vi "Auto_Routine_StraightTwoPiece.vi"(8 "error in (no error)":errorcluster) -> (0 "error out":errorcluster)   [LabVIEW 2023]
uses:
  Arm2/ArmGetSetpointEnum.ctl
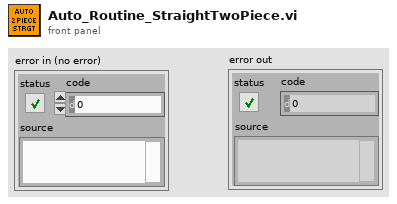
[diagram p1: front panel]
types:
  T1 = typedef "ArmGetSetpointEnum.ctl" = enum16{"ArmFloorPickup", "ArmAmpDeposit", "ArmSpeakerShoot", "ArmStartPosition", "ArmRestPosition", "ArmSourceIntake", "ArmAwayShoot"}
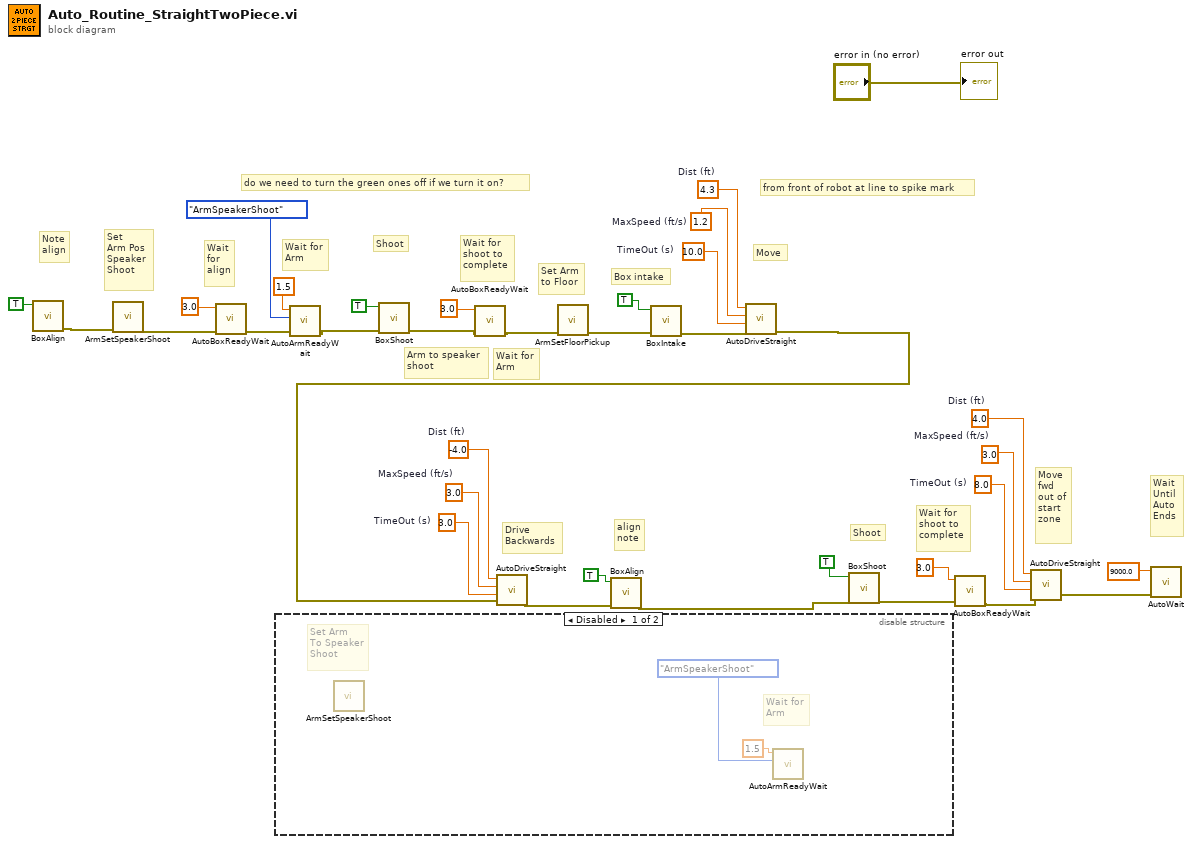
[diagram p0: block diagram]
diagram:
  w33 = 8.0  # TimeOut (s)
  w32 = 3.0  # MaxSpeed (ft/s)
  w31 = 4.0  # Dist (ft)
  w28 = 3.0  # TimeOut (s)
  w27 = 3.0  # MaxSpeed (ft/s)
  w26 = -4.0  # Dist (ft)
  w14 = 10.0  # TimeOut (s)
  w13 = 1.2  # MaxSpeed (ft/s)
  w12 = 4.3  # Dist (ft)
  # "Wait\nfor\nalign"
  # "Note\nalign"
  # "align\nnote"
  # "Wait\nUntil\nAuto \nEnds"
  # "Move\nfwd\nout of\nstart\nzone"
  # "Wait for\nshoot to\ncomplete"
  # "Shoot"
  # "Drive\nBackwards"
  # "Wait for\nArm"
  # "Arm to speaker\nshoot"
  # "Box intake"
  # "Move"
  # "Set Arm\nto Floor"
  # "Wait for\nshoot to\ncomplete"
  # "Shoot"
  # "Wait for\nArm"
  # "Set\nArm Pos\nSpeaker\nShoot"
  # "do we need to turn the green ones off if we turn it on?"
  # "from front of robot at line to spike mark"
  n1 = call "BoxAlign.vi"("box align"=TRUE) -> ("error out"=w9:errorcluster)  [unwired: 10 in]
  n2 = call "ArmSetSpeakerShoot.vi"("error in (no error)"=w9) -> ("error out"=w6:errorcluster)  [unwired: 10 in]
  n3 = call "AutoBoxReadyWait.vi"("error in (no error)"=w6, "TimeOut (s)"=3.0) -> ("error out"=w5:errorcluster)  [unwired: 9 in]
  n4 = disable-structure shown="Disabled" {
    frame Disabled {
      # "Wait for\nArm"
      # "Set Arm\nTo Speaker\nShoot"
      n5 = call "ArmSetSpeakerShoot.vi"() -> ()  [unwired: 11 in, 1 out]
      n6 = call "AutoArmReadyWait.vi"("ArmSetpoints"=ArmGetSetpointEnum."ArmSpeakerShoot", "TimeOut (s)"=1.5) -> ("error in (no error)"=w36:errorcluster)  [unwired: 8 in, 1 out]
    }
    frame Enabled {
    }
  }
  n7 = call "AutoArmReadyWait.vi"("error in (no error)"=w5, "ArmSetpoints"=ArmGetSetpointEnum."ArmSpeakerShoot", "TimeOut (s)"=1.5) -> ("error out"=w20:errorcluster)  [unwired: 8 in]
  n8 = call "BoxShoot.vi"("error in (no error)"=w20, "Box shoot"=TRUE) -> ("error out"=w22:errorcluster)  [unwired: 9 in]
  n9 = call "AutoBoxReadyWait.vi"("error in (no error)"=w22, "TimeOut (s)"=3.0) -> ("error out"=w23:errorcluster)  [unwired: 9 in]
  n10 = call "ArmSetFloorPickup.vi"("error in (no error)"=w23) -> ("error out"=w18:errorcluster)  [unwired: 10 in]
  n11 = call "BoxIntake.vi"("error in (no error)"=w18, "Box intake"=TRUE) -> ("error out"=w19:errorcluster)  [unwired: 9 in]
  n12 = call "AutoDriveStraight.vi"("error in (no error)"=w19, "TimeOut (s)"=w14, "MaxSpeed (ft/s)"=w13, "Dist (ft)"=w12) -> ("error out"=w2:errorcluster)  [unwired: 7 in]
  n13 = call "AutoDriveStraight.vi"("error in (no error)"=w2, "TimeOut (s)"=w28, "MaxSpeed (ft/s)"=w27, "Dist (ft)"=w26) -> ("error out"=w3:errorcluster)  [unwired: 7 in]
  n14 = call "BoxAlign.vi"("error in (no error)"=w3, "box align"=TRUE) -> ("error out"=w1:errorcluster)  [unwired: 9 in]
  n15 = call "BoxShoot.vi"("error in (no error)"=w1, "Box shoot"=TRUE) -> ("error out"=w29:errorcluster)  [unwired: 9 in]
  n16 = call "AutoBoxReadyWait.vi"("error in (no error)"=w29, "TimeOut (s)"=3.0) -> ("error out"=w34:errorcluster)  [unwired: 9 in]
  n17 = call "AutoDriveStraight.vi"("error in (no error)"=w34, "TimeOut (s)"=w33, "MaxSpeed (ft/s)"=w32, "Dist (ft)"=w31) -> ("error out"=w35:errorcluster)  [unwired: 7 in]
  n18 = call "AutoWait.vi"("error in (no error)"=w35, "TimeOut (s)"=9000.0) -> ()  [unwired: 9 in, 1 out]
  "error out" <- "error in (no error)"
